vi "Change Structure of Filter.vi"() -> ()   [LabVIEW 2023]
doc: "Demonstrates how to use the DFD Convert Structure VI to convert a filter to a specified structure and how to use the DFD Get Filter Structure VI to get the structure of a filter. \n\nComplete the following steps to use this VI.\n1) Run the VI.\n2) Observe the Current Structure output. \n3) Change the <B>New Structure</B> input to another infinite impulse response (IIR) filter structure.\n4) Observe the Current Structure output, which returns the same filter structure that you specified in the <B>New Structure</B> input.\n5) Change the <B>New Structure</B> input to a structure other than an IIR filter structure, for example FIR Direct Form.\n6) Observe the Current Structure output, which does not return the new structure that you specified, and the Error Message output.\n7) Click the <B>STOP</B> button to stop this VI.\n7) Examine the block diagram of this VI to learn how to use the DFD Convert Structure VI and the DFD Get Filter Structure VI."
uses:
  <vilib>/addons/Digital Filter Design/NI_DigFilterLicensed.lvlib
panel:
  in  "New Structure":u16(ring)=12 items=["FIR Direct Form"=1, "FIR Direct Form Transposed"=2, "FIR Symmetric"=3, "FIR Antisymmetric"=4, "IIR Direct Form I"=5, "IIR Direct Form I Transposed"=6, "IIR Direct Form II"=7, "IIR Direct Form II Transposed"=8, "IIR Cascaded Second-Order Sections Form I"=9, "IIR Cascaded Second-Order Sections Form I Transposed"=10, "IIR Cascaded Second-Order Sections Form II"=11, "IIR Cascaded Second-Order Sections Form II Transposed"=12, "Lattice Allpass (basic sections)"=13, "Lattice Allpass (one multiplier sections)"=14, "Lattice Allpass (normalized sections)"=15, "Lattice AR (basic sections)"=16, "Lattice AR (one multiplier sections)"=17, "Lattice AR (normalized sections)"=18, "Lattice MA (minimum phase)"=19, "Lattice MA (maximum phase)"=20, "Lattice ARMA (basic sections)"=21, "Lattice ARMA (one multiplier sections)"=22, "Lattice ARMA (normalized sections)"=23]
  out "Current Structure":u16(ring)=12 items=["Invalid", "FIR Direct Form", "FIR Direct Form Transposed", "FIR Symmetric", "FIR Antisymmetric", "IIR Direct Form I", "IIR Direct Form I Transposed", "IIR Direct Form II", "IIR Direct Form II Transposed", "IIR Cascaded Second-Order Sections Form I", "IIR Cascaded Second-Order Sections Form I Transposed", "IIR Cascaded Second-Order Sections Form II", "IIR Cascaded Second-Order Sections Form II Transposed", "Lattice Allpass (basic sections)", "Lattice Allpass (one multiplier sections)", "Lattice Allpass (normalized sections)", "Lattice AR (basic sections)", "Lattice AR (one multiplier sections)", "Lattice AR (normalized sections)", "Lattice MA (minimum phase)", "Lattice MA (maximum phase)", "Lattice ARMA (basic sections)", "Lattice ARMA (one multiplier sections)", "Lattice ARMA (normalized sections)"]
  in  "stop":bool
  out "Error Message":string
  # "Select Help>>Show Context Help and move the cursor over the VI icon for more information."
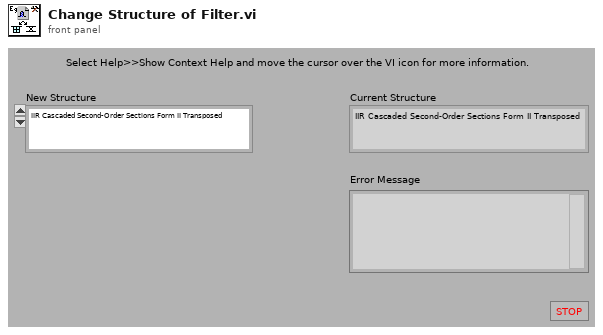
[diagram p1: front panel]
types:
  T1 = typedef "NI_DigFilterLicensed.lvlib/DFD Filter Obj.ctl" = cluster{"mSRate_Fs":dbl, "mSRate_Version":string, "mSRate_Comments":string, "mSRate_OrgCoef":T2, "mSRate_CurCoef":T2, "mSRate_Quantized?":bool, "mSRate_QCoef":T2, "mSRate_QSettings":T4[], "mSRate_Order":i32, "mSRate_Scaling":cluster{"mSRate_ScaleByPowerOf2?":bool, "mSRate_ScaleType":T6}}
  T2 = typedef "NI_DigFilterLicensed.lvlib/DFD Filter Coef.ctl" = cluster{"type":T3, "gain":dbl, "coef a (k)":dbl[], "coef b (v)":dbl[]}
  T3 = typedef "NI_DigFilterLicensed.lvlib/DFD Filter Structure Type Selector.ctl" = enum16{"Undefined", "FIR Direct Form", "FIR Direct Form Transposed", "FIR Symmetric", "FIR Antisymmetric", "IIR Direct Form I", "IIR Direct Form I Transposed", "IIR Direct Form II", "IIR Direct Form II Transposed", "IIR Cascaded Second Order Sections Form I", "IIR Cascaded Second Order Sections Form I Transposed", "IIR Cascaded Second Order Sections Form II", "IIR Cascaded Second Order Sections Form II Transposed", "Lattice Allpass (basic sections)", "Lattice Allpass (one multiplier sections)", "Lattice Allpass (normalized sections)", "Lattice AR (basic sections)", "Lattice AR (one multiplier sections)", "Lattice AR (normalized sections)", "Lattice MA (minimum phase)", "Lattice MA (maximum phase)", "Lattice ARMA (basic sections)", "Lattice ARMA (one multiplier sections)", "Lattice ARMA (normalized sections)"}
  T4 = typedef "NI_DigFilterLicensed.lvlib/dfd_Internal Quantization Settings.ctl" = cluster{"source":T5, "wl":i16, "iwl":i16, "overflow mode":enum16{"Saturation", "Wrap"}, "rounding mode":enum16{"Nearest", "Truncation"}, "signed?":bool}
  T5 = typedef "NI_DigFilterLicensed.lvlib/dfd_Internal Quantization Srcs.ctl" = u16
  T6 = typedef "NI_DigFilterLicensed.lvlib/DFD Coef Norm Type.ctl" = enum16{"No Norm", "Time Domain 1-Norm", "Time Domain 2-Norm", "Time Domain Inf-Norm"}
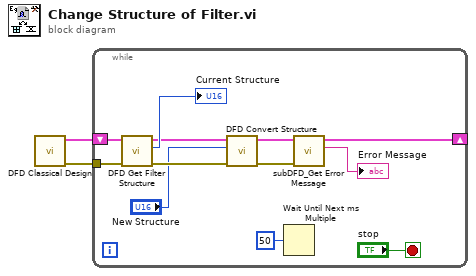
[diagram p0: block diagram]
diagram:
  n1 = call <vilib>:"DFD Classical Design.vi"() -> ("error out"=w1:errorcluster, "filter out"=w2:T1)  [unwired: 6 in, 4 out]
  n2 = while {
    tunnel: w1 -> [w12]
    shift-right: [w8] -> _
    shift-left: w2 -> [w13]
    stop <- "stop" stop-if-true
    n3 = call <vilib>:"DFD Get Filter Structure.vi"("error in (no error)"=w12, "filter in"=w13) -> ("error out"=w9:errorcluster, "structure"=→"Current Structure":u16, "filter out"=w10:T1)  [unwired: 7 out]
    n4 = call <vilib>:"DFD Convert Structure.vi"("error in (no error)"=w9, "target structure"="New Structure", "filter in"=w10) -> ("error out"=w4:errorcluster, "filter out"=w8:T1)  [unwired: 7 out]
    n5 = Wait Until Next ms Multiple(millisecond multiple=u32 50) -> ()  [unwired: 1 out]
    n6 = call <vilib>:"subDFD_Get Error Message.vi"("error in (no error)"=w4) -> ("Error Message"=→"Error Message":string)  [unwired: 10 out]
  }
